vi "Show Core Error Notification.vi"(10 "Error VIs":string[](array[string])) -> ()   [LabVIEW 2020, in "Monitored Actor.lvlib" / "Classic Monitor.lvclass"]
doc: "Displays a one button dialog with the list of Actor cores that couldn't be opened\n\nCopyright: MGI 2016\nAuthor: Derek Trepanier"
uses:
  <vilib>/MGI/Monitored Actor/Classic Monitor/Monitor/Monitor Actor/Classic Monitor.lvclass
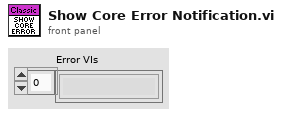
[diagram p1: front panel]
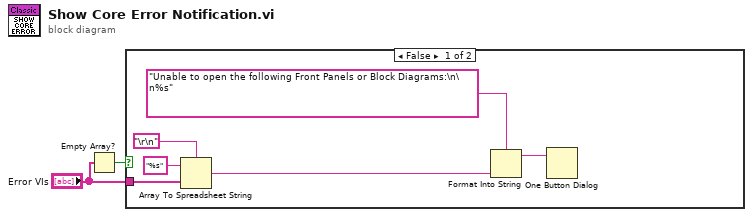
[diagram p0: block diagram]
diagram:
  n1 = Empty Array?(array="Error VIs") -> (empty?=w2:bool)
  n2 = case shown="False" w2 {
    tunnel: "Error VIs" -> [w8 _]
    frame False {
      n3 = Array To Spreadsheet String(delimiter (Tab)="\r\n", array=w8, 3:"%s" ("format string")) -> (spreadsheet string=w4:string)
      n4 = Format Into String(format string="Unable to open the following Front Panels or Block Diagrams:\n\n%s", w4) -> (resulting string=w3:string)  [unwired: 2 in, 1 out]
      n5 = One Button Dialog(message=w3) -> ()  [unwired: 1 in, 1 out]
    }
    frame True {
    }
  }
